vi "Read Write Signals Wrapper.vi"   [LabVIEW 2015]
uses:
  <vilib>/LV-Signals/read-write-xnode/LV-Read-Write-Signals.xnode
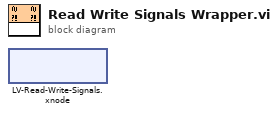
[diagram p0: block diagram]
diagram:
  n1 = xnode "LV-Read-Write-Signals.xnode"() -> ()  [unwired: 2 in, 3 out]
